vi "main.vi"() -> ()   [LabVIEW 2020, in "mainLibrary.lvlib"]
uses:
  mainLibrary.lvlib
panel:
  in  "laserSensor 3":bool
  in  "laserSensor 2":bool
  in  "laserSensor 1":bool
  out "Live View":T1(plugin-control)
  out "username":string
  in  "setting":bool
  out "softwareName":string="DORSA Palletcar Inspection System (DPIS)"
  out "timeDate":string="2024/02/02  23:23:23"
  in  "maintenance":bool
  in  "shutdown":bool
  in  "restart":bool
  in  "close":bool
  in  "report":bool
  in  "login":bool=TRUE
  out "pallet 124":bool
  out "pallet 123":bool
  out "pallet 122":bool
  out "pallet 121":bool
  out "pallet 120":bool
  out "pallet 119":bool
  out "pallet 118":bool
  out "pallet 117":bool
  out "pallet 116":bool
  out "pallet 115":bool
  out "pallet 114":bool
  out "pallet 113":bool
  out "pallet 112":bool
  out "pallet 111":bool
  out "pallet 110":bool
  out "pallet 109":bool
  out "pallet 108":bool
  out "pallet 107":bool
  out "pallet 106":bool
  out "pallet 105":bool
  out "pallet 104":bool
  out "pallet 103":bool
  out "pallet 102":bool
  out "pallet 101":bool
  out "pallet 100":bool
  out "pallet 99":bool
  out "pallet 98":bool
  out "pallet 97":bool
  out "pallet 96":bool
  out "pallet 95":bool
  out "pallet 94":bool
  out "pallet 93":bool
  out "pallet 92":bool
  out "pallet 91":bool
  out "pallet 90":bool
  out "pallet 89":bool
  out "pallet 88":bool
  out "pallet 87":bool
  out "pallet 86":bool
  out "pallet 85":bool
  out "pallet 84":bool
  out "pallet 83":bool
  out "pallet 82":bool
  out "pallet 81":bool
  out "pallet 80":bool
  out "pallet 79":bool
  out "pallet 78":bool
  out "pallet 77":bool
  out "pallet 76":bool
  out "pallet 75":bool
  out "pallet 74":bool
  out "pallet 73":bool
  out "pallet 72":bool
  out "pallet 71":bool
  out "pallet 70":bool
  out "pallet 69":bool
  out "pallet 68":bool
  out "pallet 67":bool
  out "pallet 66":bool
  out "pallet 65":bool
  out "pallet 64":bool
  out "pallet 63":bool
  out "pallet 62":bool
  out "pallet 61":bool
  out "pallet 60":bool
  out "pallet 59":bool
  out "pallet 58":bool
  out "pallet 57":bool
  out "pallet 56":bool
  out "pallet 55":bool
  out "pallet 54":bool
  out "pallet 53":bool
  out "pallet 52":bool
  out "pallet 51":bool
  out "pallet 50":bool
  out "pallet 49":bool
  out "pallet 48":bool
  out "pallet 47":bool
  out "pallet 46":bool
  out "pallet 45":bool
  out "pallet 44":bool
  out "pallet 43":bool
  out "pallet 42":bool
  out "pallet 41":bool
  out "pallet 40":bool
  out "pallet 39":bool
  out "pallet 38":bool
  out "pallet 37":bool
  out "pallet 36":bool
  out "pallet 35":bool
  out "pallet 34":bool
  out "pallet 33":bool
  out "pallet 32":bool
  out "pallet 31":bool
  out "pallet 30":bool
  out "pallet 29":bool
  out "pallet 28":bool
  out "pallet 27":bool
  out "pallet 26":bool
  out "pallet 25":bool
  out "pallet 24":bool
  out "pallet 23":bool
  out "pallet 22":bool
  out "pallet 21":bool
  out "pallet 20":bool
  out "pallet 19":bool
  out "pallet 18":bool
  out "pallet 17":bool
  out "pallet 16":bool
  out "pallet 15":bool
  out "pallet 14":bool
  out "pallet 13":bool
  out "pallet 12":bool
  out "pallet 11":bool
  out "pallet 10":bool
  out "pallet 9":bool
  out "pallet 8":bool
  out "pallet 7":bool
  out "pallet 6":bool
  out "pallet 5":bool
  out "pallet 4":bool
  out "pallet 3":bool
  out "pallet 2":bool
  out "pallet 1":bool
  out "pallet 248":bool
  out "pallet 247":bool
  out "pallet 246":bool
  out "pallet 245":bool
  out "pallet 244":bool
  out "pallet 243":bool
  out "pallet 242":bool
  out "pallet 241":bool
  out "pallet 240":bool
  out "pallet 239":bool
  out "pallet 238":bool
  out "pallet 237":bool
  out "pallet 236":bool
  out "pallet 235":bool
  out "pallet 234":bool
  out "pallet 233":bool
  out "pallet 232":bool
  out "pallet 231":bool
  out "pallet 230":bool
  out "pallet 229":bool
  out "pallet 228":bool
  out "pallet 227":bool
  out "pallet 226":bool
  out "pallet 225":bool
  out "pallet 224":bool
  out "pallet 223":bool
  out "pallet 222":bool
  out "pallet 221":bool
  out "pallet 220":bool
  out "pallet 219":bool
  out "pallet 218":bool
  out "pallet 217":bool
  out "pallet 216":bool
  out "pallet 215":bool
  out "pallet 214":bool
  out "pallet 213":bool
  out "pallet 212":bool
  out "pallet 211":bool
  out "pallet 210":bool
  out "pallet 209":bool
  out "pallet 208":bool
  out "pallet 207":bool
  out "pallet 206":bool
  out "pallet 205":bool
  out "pallet 204":bool
  out "pallet 203":bool
  out "pallet 202":bool
  out "pallet 201":bool
  out "pallet 200":bool
  out "pallet 199":bool
  out "pallet 198":bool
  out "pallet 197":bool
  out "pallet 196":bool
  out "pallet 195":bool
  out "pallet 194":bool
  out "pallet 193":bool
  out "pallet 192":bool
  out "pallet 191":bool
  out "pallet 190":bool
  out "pallet 189":bool
  out "pallet 188":bool
  out "pallet 187":bool
  out "pallet 186":bool
  out "pallet 185":bool
  out "pallet 184":bool
  out "pallet 183":bool
  out "pallet 182":bool
  out "pallet 181":bool
  out "pallet 180":bool
  out "pallet 179":bool
  out "pallet 178":bool
  out "pallet 177":bool
  out "pallet 176":bool
  out "pallet 175":bool
  out "pallet 174":bool
  out "pallet 173":bool
  out "pallet 172":bool
  out "pallet 171":bool
  out "pallet 170":bool
  out "pallet 169":bool
  out "pallet 168":bool
  out "pallet 167":bool
  out "pallet 166":bool
  out "pallet 165":bool
  out "pallet 164":bool
  out "pallet 163":bool
  out "pallet 162":bool
  out "pallet 161":bool
  out "pallet 160":bool
  out "pallet 159":bool
  out "pallet 158":bool
  out "pallet 157":bool
  out "pallet 156":bool
  out "pallet 155":bool
  out "pallet 154":bool
  out "pallet 153":bool
  out "pallet 152":bool
  out "pallet 151":bool
  out "pallet 150":bool
  out "pallet 149":bool
  out "pallet 148":bool
  out "pallet 147":bool
  out "pallet 146":bool
  out "pallet 145":bool
  out "pallet 144":bool
  out "pallet 143":bool
  out "pallet 142":bool
  out "pallet 141":bool
  out "pallet 140":bool
  out "pallet 139":bool
  out "pallet 138":bool
  out "pallet 137":bool
  out "pallet 136":bool
  out "pallet 135":bool
  out "pallet 134":bool
  out "pallet 133":bool
  out "pallet 132":bool
  out "pallet 131":bool
  out "pallet 130":bool
  out "pallet 129":bool
  out "pallet 128":bool
  out "pallet 127":bool
  out "pallet 126":bool
  out "pallet 125":bool
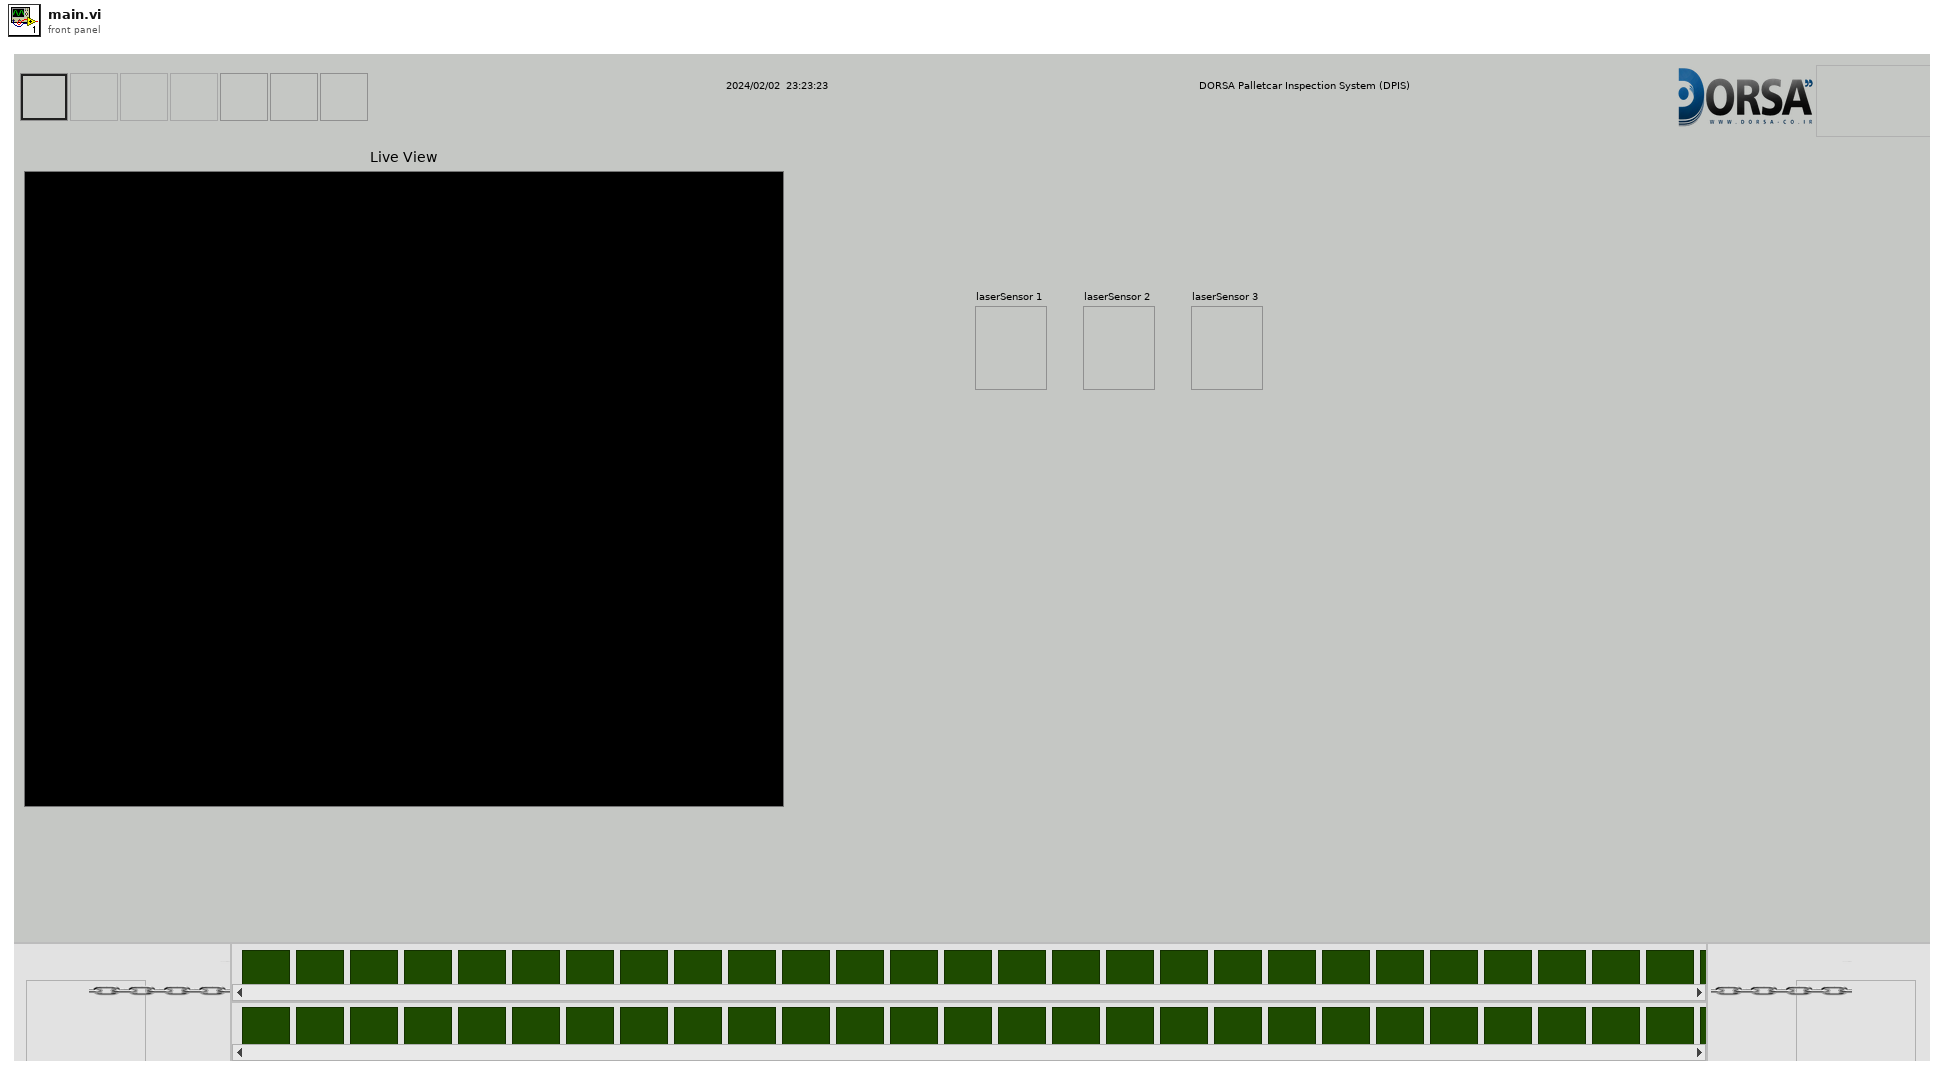
[diagram p1: front panel]
types:
  T1 = typedef "IMAQ Image.ctl" = refnum<image>
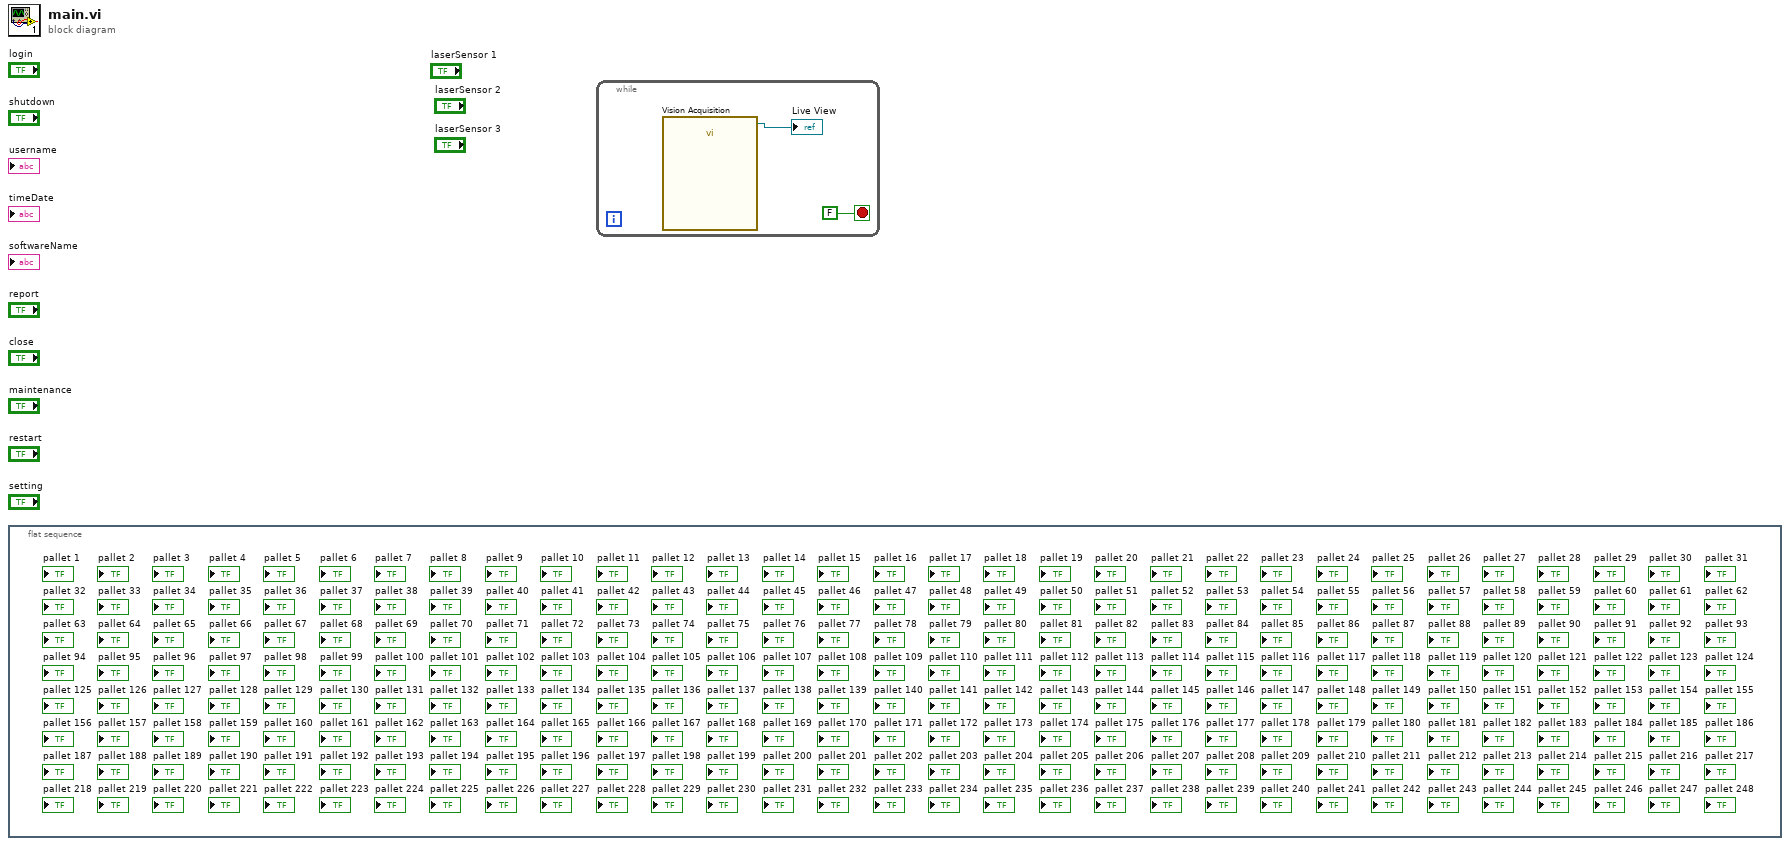
[diagram p0: block diagram]
diagram:
  n1 = flat-sequence {
    frame #0 {
    }
  }
  n2 = while {
    stop <- FALSE stop-if-true
    n3 = call "Vision Acquisition"() -> ("Image Out"=→"Live View":T1)  [unwired: 25 in, 2 out]
  }
